vi "_TangoGroupReadAttributes.vi"(2 "error in":errorcluster, 3 "attribute names":string[](array[string]), 4 "group id":i32) -> (0 "error out":errorcluster, 1 "values":T1(array[cluster]))   [LabVIEW 2014, in "tango.lvlib"]
uses:
  tango.lvlib
  tango_binding.so
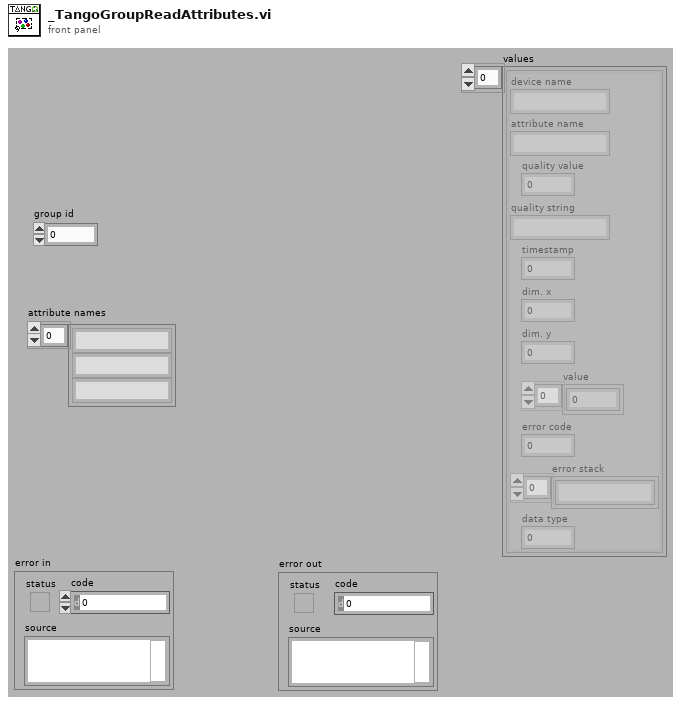
[diagram p1: front panel]
types:
  T1 = cluster{"device name":string, "attribute name":string, "quality value":i16, "quality string":string, "timestamp":dbl, "dim. x":i32, "dim. y":i32, "value":u8[], "error code":i32, "error stack":string[], "data type":u16}[]
  T2 = typedef "tango.lvlib/_AttributeValue_t.ctl" = cluster{"device name":string, "attribute name":string, "quality value":T3, "quality string":string, "timestamp":dbl, "dim. x":i32, "dim. y":i32, "value":u8[], "error code":i32, "error stack":string[], "data type":T4}
  T3 = typedef "tango.lvlib/_AttributeQuality_t.ctl" = enum16{"VALID", "INVALID", "ALARM", "CHANGING", "UNKNOWN_QUALITY"}
  T4 = typedef "tango.lvlib/_AttributeDataType_t.ctl" = enum16{"STATE_SCA", "STATE_SPE", "STATE_IMG", "STRING_SCA", "STRING_SPE", "STRING_IMG", "BOOL_SCA", "BOOL_SPE", "BOOL_IMG", "UCHAR_SCA", "UCHAR_SPE", "UCHAR_IMG", "SHORT_SCA", "SHORT_SPE", "SHORT_IMG", "USHORT_SCA", "USHORT_SPE", "USHORT_IMG", "LONG_SCA", "LONG_SPE", "LONG_IMG", "ULONG_SCA", "ULONG_SPE", "ULONG_IMG", "LONG64_SCA", "LONG64_SPE", "LONG64_IMG", "ULONG64_SCA", "ULONG64_SPE", "ULONG64_IMG", "FLOAT_SCA", "FLOAT_SPE", "FLOAT_IMG", "DOUBLE_SCA", "DOUBLE_SPE", "DOUBLE_IMG", "UNKNOWN_DATA_TYPE"}
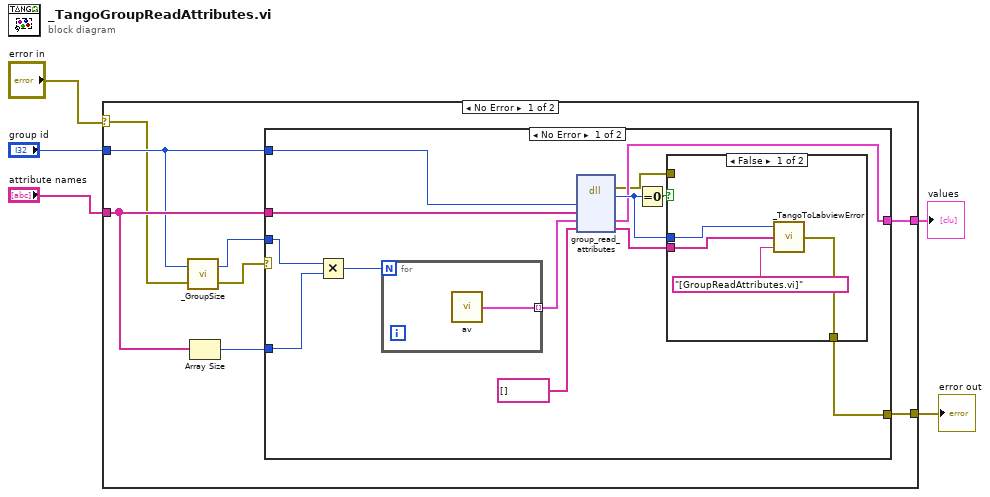
[diagram p0: block diagram]
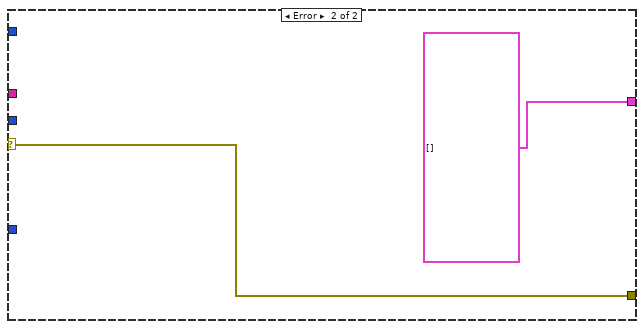
[diagram p3: hidden frame]
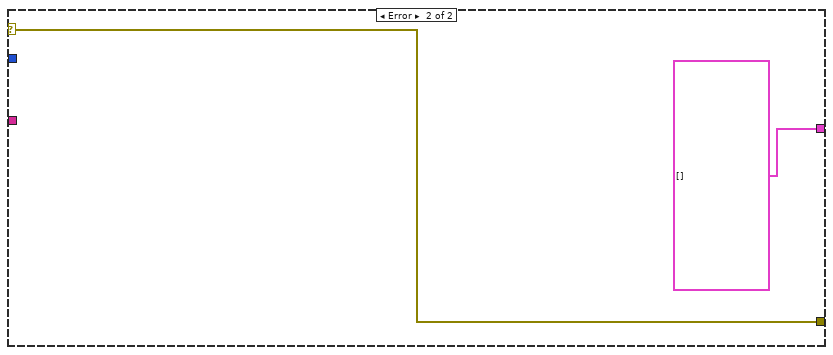
[diagram p4: hidden frame]
diagram:
  n1 = case shown="No Error" "error in" {
    selector: "error in" -> [w6 w36]
    tunnel: "group id" -> [w7 _]
    tunnel: "attribute names" -> [w13 _]
    tunnel: [w11 T1 []] -> w1
    tunnel: [w10 w36] -> w3
    frame No Error {
      n2 = call "_GroupSize.vi"("error in"=w6, "group id"=w7) -> ("error out"=w8:errorcluster, "size"=w9:i32)
      n3 = Array Size(array=w13) -> (size(s)=w12:i32)
      n4 = case shown="No Error" w8 {
        selector: w8 -> [_ w34]
        tunnel: w7 -> [w25 _]
        tunnel: w13 -> [w22 _]
        tunnel: w12 -> [w21 _]
        tunnel: [w16 T1 []] -> w11
        tunnel: [w17 w34] -> w10
        tunnel: w9 -> [w14 _]
        frame No Error {
          n5 = Multiply(x=w14, y=w21) -> (x*y=w24:i32)
          n6 = for {
            N: w24 -> [_]
            tunnel: [w32] -> w23 mode=indexing
            n7 = call "av.vi"() -> ("attribute value"=w32:T2)  [unwired: 6 in]
          }
          n8 = dll-call lib="tango_binding.*" fn="group_read_attributes"("group_id"=w25, "attribute_names"=w22, "attributes_values"=w23, "error_stack"=string[] [] ("error stack")) -> (error out=w15:errorcluster, "type de retour"=w18:i32, "attributes_values"=w16:T2[], "error_stack"=w19:string[])  [unwired: 5 in, 1 out]
          n9 = Equal To 0?(x=w18) -> (x = 0?=w20:bool)
          n10 = case shown="False" w20 {
            tunnel: w19 -> [w27 _]
            tunnel: w18 -> [w28 _]
            tunnel: [w30 w31] -> w17
            tunnel: w15 -> [_ w31]
            frame False {
              n11 = call "_TangoToLabviewError.vi"("location"="[GroupReadAttributes.vi]", "error stack"=w27, "error code"=w28) -> ("error out"=w30:errorcluster)
            }
            frame True {
            }
          }
        }
        frame Error {
        }
      }
    }
    frame Error {
    }
  }
  "error out" <- w3
  "values" <- w1
